vi "Configure SMU Output Impedance.vi"(8 "error in (no error)":errorcluster {"code" format="%.0x"}, 9 "Output Impedance (0: High)":i32(ring) items=["High", "Low"], 10 "Channel Name (1)":string="1", 11 "VISA resource name":refnum<visa-resource-name>) -> (0 "error out":errorcluster {"code" format="%.0x"}, 3 "VISA resource name out":refnum<visa-resource-name>)   [LabVIEW 2014, in "Agilent N6700 Series.lvlib"]
doc: "Specifies the output impedance mode at turn-off.\n\n<b>Note:</b>\nThis VI only applies to models N678xA SMU."
uses:
  Agilent N6700 Series.lvlib
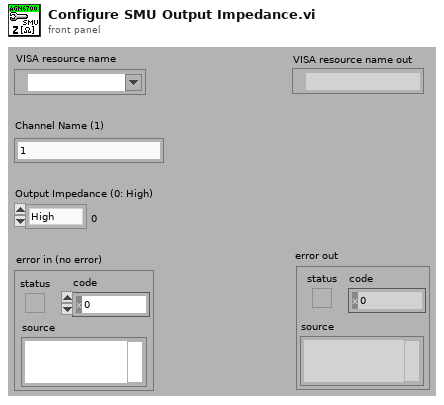
[diagram p1: front panel]
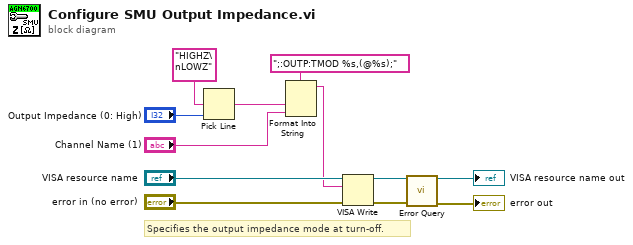
[diagram p0: block diagram]
diagram:
  # "Specifies the output impedance mode at turn-off."
  n1 = Pick Line(multi-line string="HIGHZ\nLOWZ", line index="Output Impedance (0: High)") -> (output string=w1:string)  [unwired: 1 in]
  n2 = Format Into String(format string=";:OUTP:TMOD %s,(@%s);", w1, "Channel Name (1)") -> (resulting string=w4:string)  [unwired: 2 in, 1 out]
  n3 = VISA Write(VISA resource name="VISA resource name", write buffer=w4, error in (no error)="error in (no error)") -> (VISA resource name out=w8:refnum<visa-resource-name>, error out=w7:errorcluster)  [unwired: 1 out]
  n4 = call "Error Query.vi"("VISA resource name"=w8, "error in (no error)"=w7) -> ("VISA resource name out"=→"VISA resource name out":refnum<visa-resource-name>, "error out"=→"error out":errorcluster)  [unwired: 10 in, 2 out]
